vi "Publish Scan Progress.vi"(8 "error in (no error)":errorcluster, 11 "Model in":refnum<class "Model.lvclass">) -> (0 "error out":errorcluster, 3 "Model out":refnum<class "Model.lvclass">)   [LabVIEW 2015, in "Model.lvclass"]
uses:
  Model.lvclass
  Typedefs/ScanProgress.ctl
  Typedefs/ActuatorSetPoints.ctl
  Typedefs/ActuatorData.ctl
  Typedefs/ToveyEngData.ctl
  Model.lvclass/Model.ctl
  User Events/User Events.lvclass/User Events.ctl
  User Events/User Events.lvclass
  Typedefs/FAMT Typedefs.lvlib
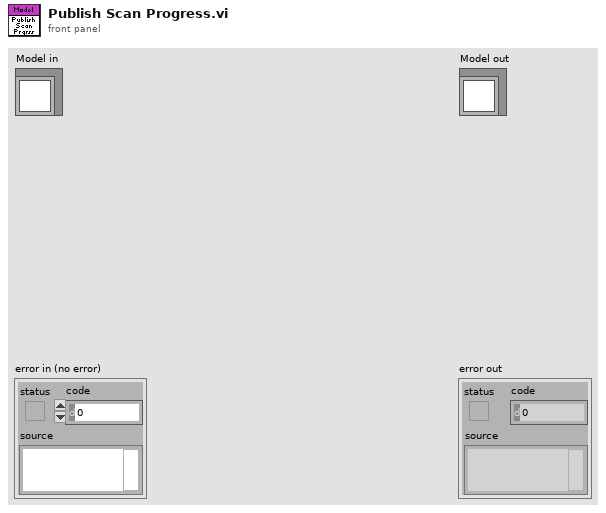
[diagram p1: front panel]
types:
  T1 = typedef "FAMT Typedefs.lvlib/ScanProgress.ctl" = cluster{"Waveform Step":u16, "Actuator Set Points":T2, "Actuator Data":T3, "Tovey Data":T4}
  T2 = typedef "FAMT Typedefs.lvlib/ActuatorSetPoints.ctl" = cluster{"Axial Force":dbl, "Lateral Force":dbl, "FC1 Force":dbl, "FC2 Force":dbl}
  T3 = typedef "FAMT Typedefs.lvlib/ActuatorData.ctl" = cluster{"Timestamp":dbl, "Axial Force":dbl, "Lateral Force":dbl, "FC1 Force":dbl, "FC2 Force":dbl, "Lateral Push Pressure":dbl, "Lateral Pull Pressure":dbl, "Axial Push Pressure":dbl, "Axial Pull Pressure":dbl}
  T4 = typedef "FAMT Typedefs.lvlib/ToveyEngData.ctl" = cluster{"Timestamp":dbl, "Fx":dbl, "Fy":dbl, "Fz":dbl, "Mx":dbl, "My":dbl, "Mz":dbl}
  T5 = typedef "FAMT Typedefs.lvlib/Publish Data Events.ctl" = cluster{"State":refnum<user-event>, "ErrorCode":refnum<user-event>, "Scan Progress":refnum<user-event>}
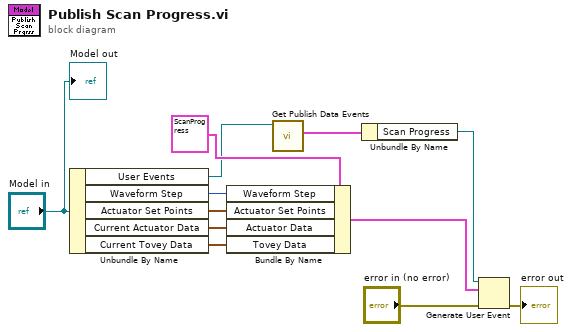
[diagram p0: block diagram]
diagram:
  n1 = Unbundle By Name("Model in") -> ("User Events"=w5:refnum<class "User Events.lvclass">, "Waveform Step"=w4:i32, "Actuator Set Points"=w3:T2, "Current Actuator Data"=w2:T3, "Current Tovey Data"=w1:T4)
  n2 = Bundle By Name(cluster=T1 {"Waveform Step"=0, "Actuator Set Points"={"Axial Force"=0.0, "Lateral Force"=0.0, "FC1 Force"=0.0, "FC2 Force"=0.0}, "Actuator Data"={"Timestamp"=0.0, "Axial Force"=0.0, "Lateral Force"=0.0, "FC1 Force"=0.0, "FC2 Force"=0.0, "Lateral Push Pressure"=0.0, "Lateral Pull Pressure"=0.0, "Axial Push Pressure"=0.0, "Axial Pull Pressure"=0.0}, "Tovey Data"={"Timestamp"=0.0, "Fx"=0.0, "Fy"=0.0, "Fz"=0.0, "Mx"=0.0, "My"=0.0, "Mz"=0.0}} ("event data"), "Waveform Step"=w4, "Actuator Set Points"=w3, "Actuator Data"=w2, "Tovey Data"=w1) -> (w7:T1)
  n3 = call "Get Publish Data Events.vi"("UserEvents in"=w5) -> ("Publish Data Events"=w11:T5)  [unwired: 9 in, 1 out]
  n4 = Unbundle By Name(w11) -> ("Scan Progress"=w12:refnum<user-event>)
  n5 = Generate User Event(user event=w12, event data cluster=w7, error in="error in (no error)") -> (error out=→"error out":errorcluster)  [unwired: 1 in, 1 out]
  "Model out" <- "Model in"
